vi "ReadUsers.vi"(4 "error in (no error)":errorcluster, 7 "configuration file path":path) -> (0 "error out":errorcluster, 2 "known users":string[](array[string]), 3 "configuration file path dup":path)   [LabVIEW 2015]
uses:
  <vilib>/Utility/config.llb/NI_LVConfig.lvlib
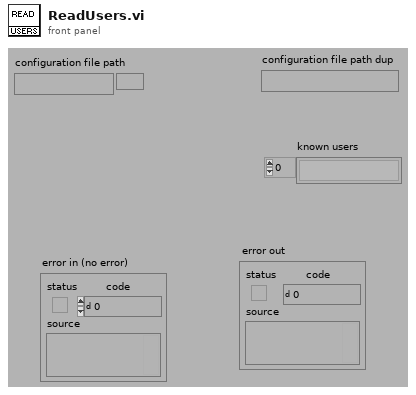
[diagram p1: front panel]
types:
  T1 = typedef "NI_LVConfig.lvlib/Config Data RefNum.ctl" = refnum<k1>
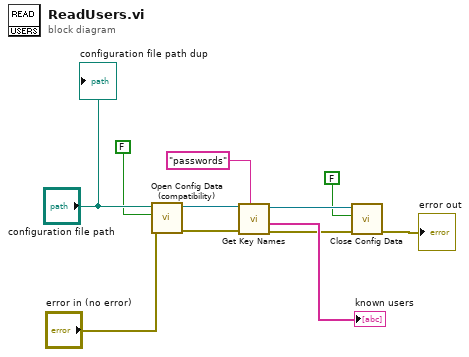
[diagram p0: block diagram]
diagram:
  n1 = call <vilib>:"Open Config Data (compatibility).vi"("error in (no error)"="error in (no error)", "create file if necessary (T)"=FALSE, "configuration file path"="configuration file path") -> ("error out"=w7:errorcluster, "refnum"=w8:T1)  [unwired: 6 in, 1 out]
  n2 = call <vilib>:"Get Key Names.vi"("section"="passwords", "error in (no error)"=w7, "refnum"=w8) -> ("error out"=w3:errorcluster, "key names"=→"known users":string[], "refnum out"=w4:T1)  [unwired: 5 in, 1 out]
  n3 = call <vilib>:"Close Config Data.vi"("error in (no error)"=w3, "write file if changed (T)"=FALSE, "refnum"=w4) -> ("error out"=→"error out":errorcluster)  [unwired: 7 in, 1 out]
  "configuration file path dup" <- "configuration file path"
